vi "CCD-PDA_Exposure.vi"(4 "Current Detector":T1, 5 "error in":errorcluster, 8 "CCD Parameters":T2={"Exposure Time (s)"=0.2, "Offset"=0.0, "BkgrdCrct"=FALSE, "Shutter"=FALSE, "Mode"=enum."Regular", "Repetition"=4, "dt or s"=0.0} {"dt or s" format="%#.6f"; "Repetition" min=1; "Offset" format="%#.2f"; "Exposure Time (s)" min=0.02 max=6000.0 format="%#.2f"}) -> (0 "Error Out":errorcluster, 1 "The Data":dbl[](array[numeric])=[1198.0, 1190.0, 1193.0, 1194.0, 1189.0, 1188.0, 1196.0, 1190.0, 1202.0, 1191.0, 1193.0, 1192.0, 1199.0, 1189.0, 1194.0, 1189.0, 1197.0, 1191.0, 1187.0, 1192.0, 1195.0, 1189.0, 1195.0, 1191.0, 1199.0, 1194.0, 1192.0, 1191.0, 1193.0, 1197.0, 1193.0, 1193.0, 1194.0, 1200.0, 1191.0, 1190.0, 1187.0, 1195.0, 1189.0, 1188.0, 1191.0, 1194.0, 1187.0, 1192.0, 1198.0, 1193.0, 1190.0, 1192.0, 1190.0, 1193.0, 1191.0, 1190.0, 1191.0, 1189.0, 1192.0, 1194.0, 1190.0, 1193.0, 1193.0, 1191.0, 1194.0, 1182.0, 1190.0, 1188.0, 1199.0, 1192.0, 1196.0, 1195.0, 1186.0, 1189.0, 1188.0, 1185.0, 1194.0, 1187.0, 1193.0, 1194.0, 1190.0, 1189.0, 1189.0, 1187.0, 1196.0, 1195.0, 1191.0, 1197.0, 1192.0, 1200.0, 1187.0, 1194.0, 1189.0, 1193.0, 1195.0, 1196.0, 1186.0, 1192.0, 1190.0, 1194.0, 1194.0, 1190.0, 1191.0, 1193.0, 1197.0, 1197.0, 1185.0, 1199.0, 1190.0, 1195.0, 1196.0, 1184.0, 1193.0, 1193.0, 1193.0, 1191.0, 1189.0, 1190.0, 1199.0, 1193.0, 1191.0, 1194.0, 1191.0, 1192.0, 1186.0, 1190.0, 1194.0, 1189.0, 1194.0, 1190.0, 1191.0, 1192.0, 1192.0, 1196.0, 1192.0, 1192.0, 1189.0, 1193.0, 1198.0, 1186.0, 1191.0, 1193.0, 1187.0, 1194.0, 1190.0, 1190.0, 1191.0, 1189.0, 1194.0, 1195.0, 1189.0, 1192.0, 1185.0, 1193.0, 1192.0, 1192.0, 1189.0, 1191.0, 1191.0, 1190.0, 1196.0, 1194.0, 1193.0, 1191.0, 1189.0, 1191.0, 1196.0, 1192.0, 1192.0, 1189.0, 1196.0, 1191.0, 1193.0, 1192.0, 1188.0, 1190.0, 1194.0, 1192.0, 1185.0, 1191.0, 1194.0, 1191.0, 1189.0, 1195.0, 1192.0, 1196.0, 1190.0, 1193.0, 1191.0, 1189.0, 1194.0, 1195.0, 1191.0, 1187.0, 1190.0, 1196.0, 1196.0, 1192.0, 1197.0, 1191.0, 1189.0, 1192.0, 1192.0, 1200.0, 1192.0, 1193.0, 1190.0, 1192.0, 1187.0, 1198.0, 1186.0, 1196.0, 1201.0, 1199.0, 1200.0, 1191.0, 1196.0, 1200.0, 1192.0, 1191.0, 1193.0, 1185.0, 1192.0, 1194.0, 1186.0, 1190.0, 1188.0, 1189.0, 1201.0, 1197.0, 1191.0, 1194.0, 1193.0, 1194.0, 1195.0, 1198.0, 1200.0, 1192.0, 1192.0, 1193.0, 1193.0, 1195.0, 1187.0, 1193.0, 1192.0, 1187.0, 1189.0, 1186.0, 1191.0, 1197.0, 1191.0, 1200.0, 1194.0, 1192.0, 1187.0, 1196.0, 1191.0, 1191.0, 1196.0, 1187.0, 1190.0, 1193.0, 1189.0, 1193.0, 1190.0, 1188.0, 1188.0, 1190.0, 1197.0, 1188.0, 1191.0, 1195.0, 1188.0, 1191.0, 1188.0, 1194.0, 1193.0, 1187.0, 1200.0, 1192.0, 1197.0, 1190.0, 1196.0, 1200.0, 1191.0, 1189.0, 1193.0, 1189.0, 1186.0, 1196.0, 1185.0, 1198.0, 1195.0, 1186.0, 1191.0, 1197.0, 1191.0, 1193.0, 1195.0, 1193.0, 1191.0, 1198.0, 1189.0, 1183.0, 1200.0, 1197.0, 1192.0, 1192.0, 1192.0, 1196.0, 1191.0, 1190.0, 1194.0, 1188.0, 1198.0, 1193.0, 1195.0, 1190.0, 1187.0, 1192.0, 1191.0, 1195.0, 1188.0, 1190.0, 1191.0, 1187.0, 1189.0, 1185.0, 1189.0, 1196.0, 1198.0, 1191.0, 1190.0, 1196.0, 1197.0, 1193.0, 1187.0, 1186.0, 1195.0, 1191.0, 1193.0, 1192.0, 1196.0, 1190.0, 1192.0, 1192.0, 1192.0, 1190.0, 1195.0, 1192.0, 1191.0, 1193.0, 1197.0, 1184.0, 1190.0, 1188.0, 1192.0, 1194.0, 1190.0, 1193.0, 1195.0, 1195.0, 1194.0, 1189.0, 1193.0, 1191.0, 1194.0, 1186.0, 1189.0, 1192.0, 1191.0, 1182.0, 1190.0, 1197.0, 1194.0, 1188.0, 1193.0, 1191.0, 1186.0, 1194.0, 1197.0, 1193.0, 1191.0, 1187.0, 1194.0, 1194.0, 1191.0, 1189.0, 1195.0, 1194.0, 1189.0, 1196.0, 1187.0, 1186.0, 1192.0, 1194.0, 1196.0, 1191.0, 1193.0, 1191.0, 1188.0, 1190.0, 1199.0, 1198.0, 1196.0, 1196.0, 1190.0, 1194.0, 1191.0, 1194.0, 1187.0, 1195.0, 1190.0, 1194.0, 1196.0, 1194.0, 1189.0, 1193.0, 1189.0, 1194.0, 1189.0, 1195.0, 1192.0, 1194.0, 1193.0, 1191.0, 1197.0, 1187.0, 1189.0, 1189.0, 1188.0, 1197.0, 1192.0, 1189.0, 1193.0, 1194.0, 1183.0, 1202.0, 1187.0, 1192.0, 1184.0, 1188.0, 1186.0, 1193.0, 1189.0, 1195.0, 1189.0, 1193.0, 1197.0, 1189.0, 1194.0, 1191.0, 1194.0, 1192.0, 1191.0, 1191.0, 1196.0, 1194.0, 1190.0, 1193.0, 1192.0, 1195.0, 1197.0, 1198.0, 1193.0, 1202.0, 1196.0, 1194.0, 1194.0, 1190.0, 1193.0, 1190.0, 1195.0, 1192.0, 1187.0, 1194.0, 1197.0, 1190.0, 1194.0, 1189.0, 1198.0, 1192.0, 1191.0, 1192.0, 1192.0, 1191.0, 1191.0, 1193.0, 1191.0, 1191.0, 1198.0, 1186.0, 1192.0, 1185.0, 1185.0, 1188.0, 1194.0, 1196.0, 1194.0, 1195.0, 1190.0, 1194.0, 1191.0, 1190.0, 1195.0, 1191.0, 1191.0, 1195.0, 1192.0, 1194.0, 1201.0, 1187.0, 1191.0, 1195.0, 1187.0, 1192.0, 1192.0, 1193.0, 1200.0, 1188.0, 1189.0, 1189.0, 1197.0, 1189.0, 1188.0, 1197.0, 1195.0, 1191.0, 1189.0, 1190.0, 1195.0, 1189.0, 1191.0, 1194.0, 1186.0, 1192.0, 1190.0, 1191.0, 1188.0, 1195.0, 1192.0, 1191.0, 1191.0, 1199.0, 1190.0, 1190.0, 1190.0, 1192.0, 1187.0, 1193.0, 1197.0, 1197.0, 1186.0, 1193.0, 1189.0, 1192.0, 1197.0, 1184.0, 1187.0, 1188.0, 1192.0, 1192.0, 1192.0, 1189.0, 1192.0, 1190.0, 1194.0, 1191.0, 1186.0, 1196.0, 1194.0, 1189.0, 1193.0, 1191.0, 1186.0, 1189.0, 1193.0, 1195.0, 1196.0, 1197.0, 1199.0, 1194.0, 1190.0, 1193.0, 1194.0, 1190.0, 1198.0, 1196.0, 1194.0, 1195.0, 1194.0, 1184.0, 1188.0, 1195.0, 1197.0, 1190.0, 1194.0, 1190.0, 1191.0, 1195.0, 1198.0, 1188.0, 1193.0, 1194.0, 1195.0, 1198.0, 1195.0, 1191.0, 1197.0, 1192.0, 1198.0, 1190.0, 1196.0, 1191.0, 1194.0, 1188.0, 1189.0, 1198.0, 1192.0, 1198.0, 1195.0, 1185.0, 1191.0, 1193.0, 1192.0, 1197.0, 1195.0, 1195.0, 1195.0, 1193.0, 1190.0, 1190.0, 1190.0, 1198.0, 1195.0, 1191.0, 1194.0, 1190.0, 1190.0, 1194.0, 1194.0, 1195.0, 1192.0, 1190.0, 1194.0, 1195.0, 1192.0, 1192.0, 1194.0, 1189.0, 1192.0, 1193.0, 1188.0, 1194.0, 1195.0, 1196.0, 1193.0, 1192.0, 1201.0, 1191.0, 1198.0, 1197.0, 1191.0, 1192.0, 1191.0, 1194.0, 1193.0, 1188.0, 1192.0, 1189.0, 1183.0, 1189.0, 1190.0, 1192.0, 1189.0, 1196.0, 1193.0, 1197.0, 1185.0, 1193.0, 1189.0, 1191.0, 1196.0, 1195.0, 1193.0, 1193.0, 1191.0, 1189.0, 1193.0, 1192.0, 1192.0, 1192.0, 1190.0, 1191.0, 1193.0, 1193.0, 1197.0, 1195.0, 1189.0, 1193.0, 1188.0, 1194.0, 1197.0, 1194.0, 1195.0, 1196.0, 1190.0, 1194.0, 1188.0, 1197.0, 1195.0, 1191.0, 1195.0, 1192.0, 1194.0, 1188.0, 1190.0, 1197.0, 1197.0, 1191.0, 1187.0, 1197.0, 1191.0, 1193.0, 1188.0, 1191.0, 1194.0, 1193.0, 1195.0, 1192.0, 1195.0, 1189.0, 1193.0, 1193.0, 1195.0, 1190.0, 1192.0, 1196.0, 1188.0, 1187.0, 1193.0, 1192.0, 1192.0, 1194.0, 1185.0, 1199.0, 1190.0, 1193.0, 1191.0, 1198.0, 1189.0, 1190.0, 1191.0, 1190.0, 1193.0, 1195.0, 1186.0, 1190.0, 1193.0, 1191.0, 1189.0, 1197.0, 1193.0, 1198.0, 1190.0, 1192.0, 1193.0, 1191.0, 1196.0, 1193.0, 1196.0, 1190.0, 1190.0, 1198.0, 1192.0, 1199.0, 1198.0, 1190.0, 1191.0, 1191.0, 1196.0, 1190.0, 1196.0, 1195.0, 1191.0, 1196.0, 1195.0, 1193.0, 1190.0, 1190.0, 1195.0, 1193.0, 1187.0, 1197.0, 1185.0, 1191.0, 1189.0, 1191.0, 1193.0, 1192.0, 1188.0, 1196.0, 1193.0, 1191.0, 1193.0, 1193.0, 1190.0, 1192.0, 1192.0, 1192.0, 1195.0, 1191.0, 1195.0, 1189.0, 1189.0, 1191.0, 1191.0, 1185.0, 1192.0, 1191.0, 1193.0, 1201.0, 1199.0, 1197.0, 1206.0, 1201.0, 1207.0, 1200.0, 1198.0, 1195.0, 1188.0, 1194.0, 1186.0, 1190.0, 1197.0, 1188.0, 1193.0, 1196.0, 1193.0, 1192.0, 1192.0, 1188.0, 1196.0, 1186.0, 1193.0, 1194.0, 1188.0, 1190.0, 1190.0, 1192.0, 1190.0, 1191.0, 1191.0, 1200.0, 1192.0, 1199.0, 1193.0, 1190.0, 1190.0, 1199.0, 1187.0, 1193.0, 1190.0, 1188.0, 1194.0, 1194.0, 1196.0, 1194.0, 1195.0, 1190.0, 1187.0, 1187.0, 1196.0, 1193.0, 1199.0, 1190.0, 1193.0, 1193.0, 1191.0, 1198.0, 1192.0, 1193.0, 1192.0, 1193.0, 1189.0, 1189.0, 1197.0, 1189.0, 1194.0, 1193.0, 1192.0, 1185.0, 1198.0, 1193.0, 1189.0, 1192.0, 1193.0, 1196.0, 1190.0, 1195.0, 1189.0, 1196.0, 1198.0, 1190.0, 1191.0, 1193.0, 1186.0, 1189.0, 1195.0, 1188.0, 1197.0, 1188.0, 1191.0, 1185.0, 1190.0, 1193.0, 1188.0, 1198.0, 1192.0, 1193.0, 1194.0, 1194.0, 1189.0, 1184.0, 1193.0, 1199.0, 1193.0, 1192.0, 1193.0, 1190.0, 1196.0, 1191.0, 1192.0, 1189.0, 1194.0, 1188.0, 1189.0, 1190.0, 1190.0, 1192.0, 1195.0, 1188.0, 1190.0, 1192.0, 1189.0, 1197.0, 1192.0, 1194.0, 1187.0, 1196.0, 1192.0, 1194.0, 1185.0, 1187.0, 1187.0, 1191.0, 1195.0, 1190.0, 1186.0, 1183.0, 1194.0, 1194.0, 1192.0, 1192.0, 1188.0, 1193.0, 1195.0, 1189.0, 1190.0, 1191.0, 1192.0, 1196.0, 1186.0, 1195.0, 1191.0, 1185.0, 1191.0, 1187.0, 1190.0, 1188.0, 1189.0, 1187.0, 1196.0, 1191.0, 1190.0, 1191.0, 1190.0, 1196.0, 1195.0, 1186.0, 1187.0, 1187.0, 1188.0, 1194.0, 1192.0, 1192.0, 1192.0, 1189.0, 1192.0, 1191.0, 1188.0, 1188.0, 1187.0, 1187.0, 1190.0, 1186.0, 1191.0, 1195.0, 1192.0, 1196.0, 1193.0, 1192.0, 1191.0, 1189.0, 1187.0, 1193.0, 1188.0, 1189.0, 1194.0, 1191.0, 1185.0, 1193.0, 1191.0, 1196.0, 1196.0, 1199.0, 1195.0, 1211.0] format="%.2f", 2 "#PixelOverflow":u32, 3 "PixelOverflow":bool)   [LabVIEW 2019]
doc: "This is the controlling VI for CCD exposures.\nIt calls the right CCD subVIs if the \"Current Experiment Status\" Exposure status is \"OK\".\nIt will also set the \"Current Experiment Status\" Exposure status \nfrom \"OK\" to \"Busy\" to \"Done\" ."
uses:
  Globals and TypeDefs/Type Definitions.llb/CCDParameter.ctt
  Globals and TypeDefs/Type Definitions.llb/ListOfDetectors.ctt
panel:
  out "Array Length":i32=1024
  out "Plot":dbl[](graph)
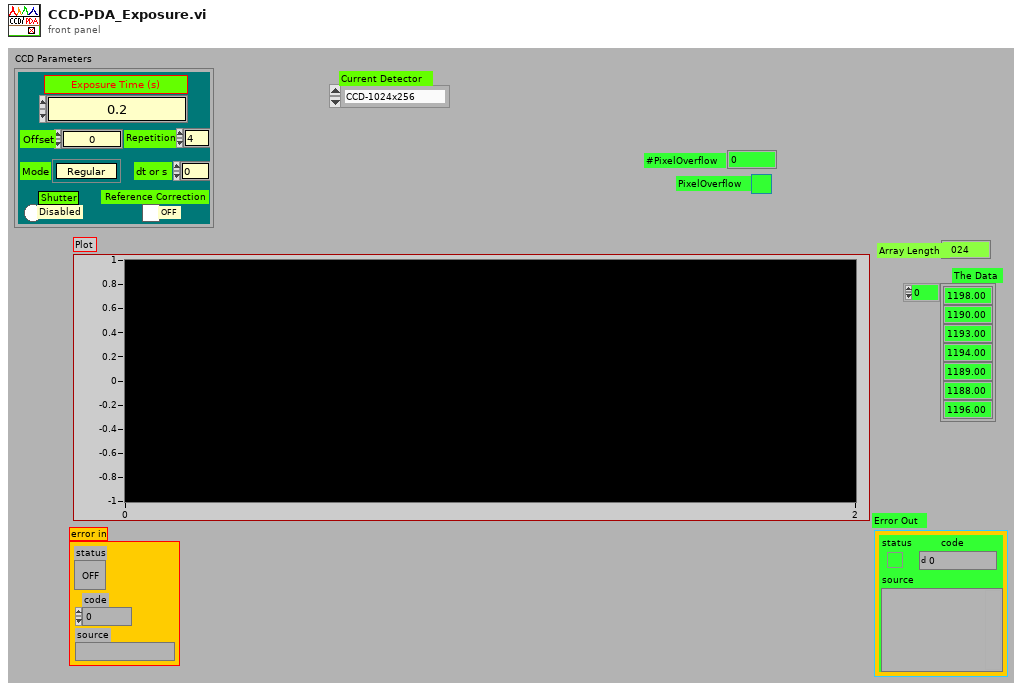
[diagram p1: front panel]
types:
  T1 = typedef "ListOfDetectors.ctt" = enum8{"CCD-1024x256", "InGaAs PDA-1024x1", "CCD-1340x400", "Ge Single Channel", "Si Single Channel", "PMT Single Channel"}
  T2 = typedef "CCDParameter.ctt" = cluster{"Exposure Time (s)":dbl, "Offset":dbl, "BkgrdCrct":bool, "Shutter":bool, "Mode":enum8{"Regular", "OverExp Cor", "SpikeRemove", "ForCalibration"}, "Repetition":u16, "dt or s":dbl}
  T3 = enum8{"Regular", "OverExp Cor", "SpikeRemove", "ForCalibration"}
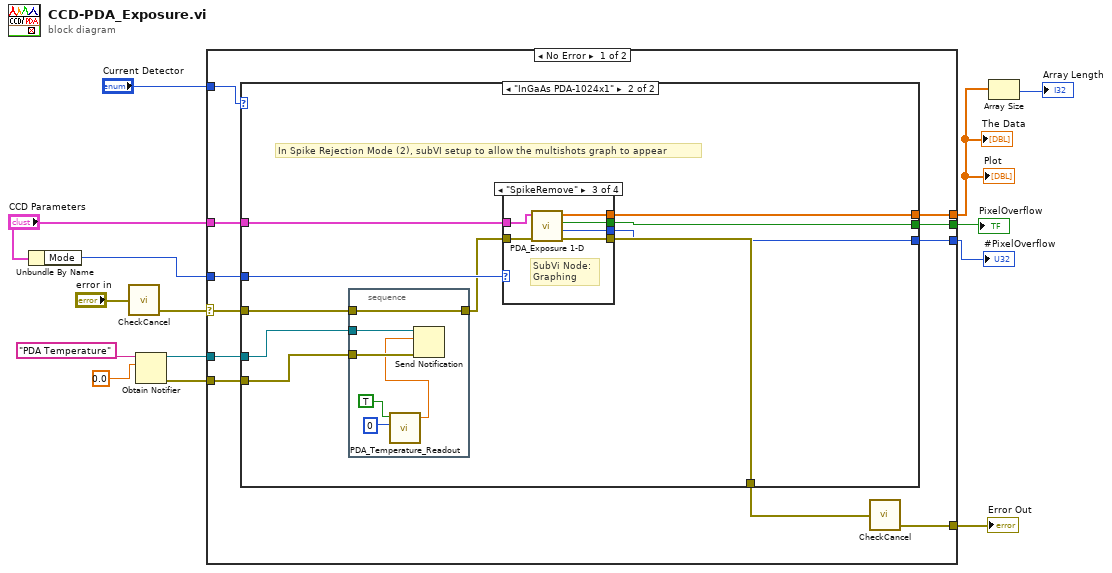
[diagram p0: block diagram]
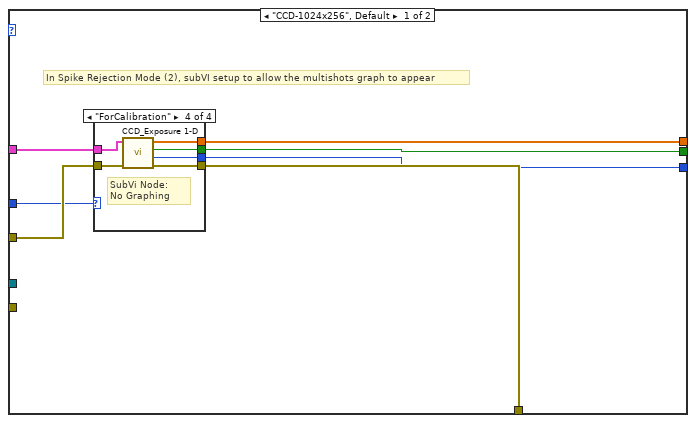
[diagram p2: hidden frame]
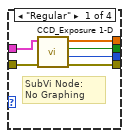
[diagram p3: hidden frame]
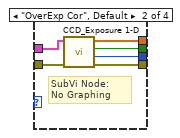
[diagram p4: hidden frame]
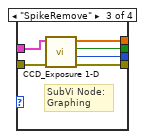
[diagram p5: hidden frame]
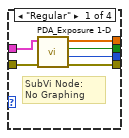
[diagram p6: hidden frame]
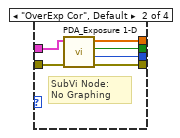
[diagram p7: hidden frame]
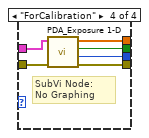
[diagram p8: hidden frame]
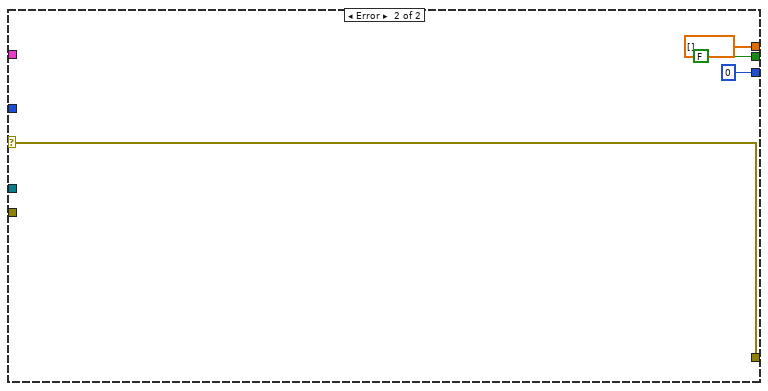
[diagram p9: hidden frame]
diagram:
  n1 = Unbundle By Name("CCD Parameters") -> ("Mode"=w5:T3)
  n2 = call "CheckCancel.vi"("error in (no error)"="error in") -> ("error out"=w6:errorcluster)  [unwired: 1 in, 1 out]
  n3 = Obtain Notifier(name (unnamed)="PDA Temperature", notification data type=0.0) -> (notifier out=w2:refnum<notifier>, error out=w1:errorcluster)  [unwired: 2 in, 1 out]
  n4 = case shown="No Error" w6 {
    selector: w6 -> [w19 w97]
    tunnel: [w18 w97] -> w14
    tunnel: "Current Detector" -> [w25 _]
    tunnel: [w24 dbl[] [] ("The Data")] -> w11
    tunnel: [w23 FALSE ("PixelOverflow")] -> w13
    tunnel: [w22 u32 0 ("#PixelOverflow")] -> w12
    tunnel: w5 -> [w21 _]
    tunnel: "CCD Parameters" -> [w20 _]
    tunnel: w2 -> [w16 _]
    tunnel: w1 -> [w15 _]
    frame No Error {
      n5 = case shown="\"InGaAs PDA-1024x1\"" w25 {
        tunnel: w19 -> [w32 w58]
        tunnel: [w31 w66] -> w17
        tunnel: [w30 w65] -> w24
        tunnel: [w29 w64] -> w23
        tunnel: [w28 w63] -> w22
        tunnel: w21 -> [w27 w62]
        tunnel: w20 -> [w26 w61]
        tunnel: w16 -> [_ w60]
        tunnel: w15 -> [_ w59]
        frame "CCD-1024x256", Default {
          # "In Spike Rejection Mode (2), subVI setup to allow the multishots graph to appear"
          n6 = case shown="\"ForCalibration\"" w27 {
            tunnel: w32 -> [w38 w44 w50 w56]
            tunnel: [w37 w43 w49 w55] -> w31
            tunnel: [w36 w42 w48 w54] -> w30
            tunnel: [w35 w41 w47 w53] -> w29
            tunnel: [w34 w40 w46 w52] -> w28
            tunnel: w26 -> [w33 w39 w45 w51]
            frame "Regular" {
              # "SubVi Node:\nNo Graphing"
              n7 = call "CCD_Exposure 1-D.vi"("error in"=w38, "CCD Parameters"=w33) -> ("Error Out"=w37:errorcluster, "#PixelOverflow"=w34:u32, "PixelOverflow"=w35:bool, "The Data"=w36:dbl[])  [unwired: 3 in, 3 out]
            }
            frame "OverExp Cor", Default {
              # "SubVi Node:\nNo Graphing"
              n8 = call "CCD_Exposure 1-D.vi"("error in"=w44, "CCD Parameters"=w39) -> ("Error Out"=w43:errorcluster, "#PixelOverflow"=w40:u32, "PixelOverflow"=w41:bool, "The Data"=w42:dbl[])  [unwired: 3 in, 3 out]
            }
            frame "SpikeRemove" {
              # "SubVi Node:\nGraphing"
              n9 = call "CCD_Exposure 1-D.vi"("error in"=w50, "CCD Parameters"=w45) -> ("Error Out"=w49:errorcluster, "#PixelOverflow"=w46:u32, "PixelOverflow"=w47:bool, "The Data"=w48:dbl[])  [unwired: 3 in, 3 out]
            }
            frame "ForCalibration" {
              # "SubVi Node:\nNo Graphing"
              n10 = call "CCD_Exposure 1-D.vi"("error in"=w56, "CCD Parameters"=w51) -> ("Error Out"=w55:errorcluster, "#PixelOverflow"=w52:u32, "PixelOverflow"=w53:bool, "The Data"=w54:dbl[])  [unwired: 3 in, 3 out]
            }
          }
        }
        frame "InGaAs PDA-1024x1" {
          # "In Spike Rejection Mode (2), subVI setup to allow the multishots graph to appear"
          n11 = stacked-sequence {
            tunnel: w60 -> [w71]
            tunnel: w59 -> [w70]
            tunnel: [w67] -> w57
            tunnel: w58 -> [w67]
            frame #0 {
              n12 = call "PDA_Temperature_Readout.vi"("stop"=TRUE, "msec to wait"=u32 0) -> ("PDA Temperature"=w69:dbl)  [unwired: 4 in, 1 out]
              n13 = Send Notification(notification=w69, notifier=w71, error in (no error)=w70) -> ()  [unwired: 2 out]
            }
          }
          n14 = case shown="\"SpikeRemove\"" w62 {
            tunnel: w57 -> [w78 w84 w90 w96]
            tunnel: [w77 w83 w89 w95] -> w66
            tunnel: [w76 w82 w88 w94] -> w65
            tunnel: [w75 w81 w87 w93] -> w64
            tunnel: [w74 w80 w86 w92] -> w63
            tunnel: w61 -> [w73 w79 w85 w91]
            frame "Regular" {
              # "SubVi Node:\nNo Graphing"
              n15 = call "PDA_Exposure 1-D.vi"("error in"=w78, "CCD Parameters"=w73) -> ("Error Out"=w77:errorcluster, "#PixelOverflow"=w74:u32, "PixelOverflow"=w75:bool, "The Data"=w76:dbl[])  [unwired: 5 in, 1 out]
            }
            frame "OverExp Cor", Default {
              # "SubVi Node:\nNo Graphing"
              n16 = call "PDA_Exposure 1-D.vi"("error in"=w84, "CCD Parameters"=w79) -> ("Error Out"=w83:errorcluster, "#PixelOverflow"=w80:u32, "PixelOverflow"=w81:bool, "The Data"=w82:dbl[])  [unwired: 5 in, 1 out]
            }
            frame "SpikeRemove" {
              # "SubVi Node:\nGraphing"
              n17 = call "PDA_Exposure 1-D.vi"("error in"=w90, "CCD Parameters"=w85) -> ("Error Out"=w89:errorcluster, "#PixelOverflow"=w86:u32, "PixelOverflow"=w87:bool, "The Data"=w88:dbl[])  [unwired: 5 in, 1 out]
            }
            frame "ForCalibration" {
              # "SubVi Node:\nNo Graphing"
              n18 = call "PDA_Exposure 1-D.vi"("error in"=w96, "CCD Parameters"=w91) -> ("Error Out"=w95:errorcluster, "#PixelOverflow"=w92:u32, "PixelOverflow"=w93:bool, "The Data"=w94:dbl[])  [unwired: 5 in, 1 out]
            }
          }
        }
      }
      n19 = call "CheckCancel.vi"("error in (no error)"=w17) -> ("error out"=w18:errorcluster)  [unwired: 1 in, 1 out]
    }
    frame Error {
    }
  }
  "Error Out" <- w14
  "The Data" <- w11
  "Plot" <- w11
  "PixelOverflow" <- w13
  "#PixelOverflow" <- w12
  n20 = Array Size(array=w11) -> (size(s)=→"Array Length":i32)
